vi "UpdateConnectionsListbox.vi"(8 "error in (no error)":errorcluster, 10 "Connections":T1[](array[typedef]), 11 "TCP_serverGUI in":refnum<class "TCP_serverGUI.lvclass">) -> (0 "error out":errorcluster, 3 "TCP_serverGUI out":refnum<class "TCP_serverGUI.lvclass">)   [LabVIEW 2023, in "TCP_serverGUI.lvlib" / "TCP_serverGUI.lvclass"]
uses:
  TCP_serverGUI.lvclass
  TCP_Listener/TypeDefinitions/ConnectionInformation.ctl
  TCP_serverGUI.lvclass/TCP_serverGUI.ctl
  TCP_Listener/TCP_Listener.lvlib
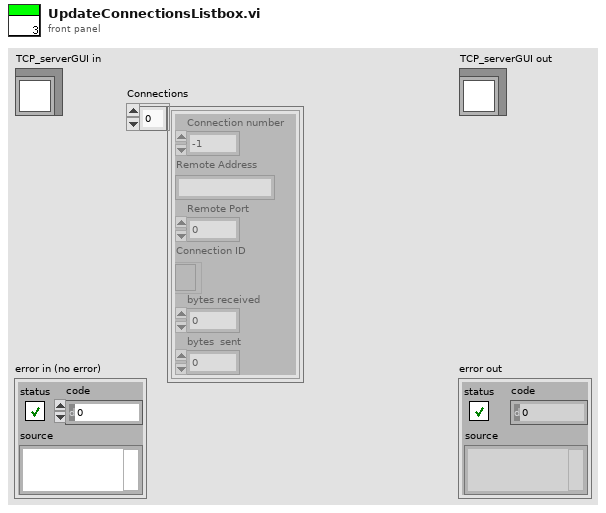
[diagram p1: front panel]
types:
  T1 = typedef "TCP_Listener.lvlib/ConnectionInformation.ctl" = cluster{"Connection number":i32, "Remote Address":string, "Remote Port":u16, "Connection ID":refnum<k5>, "bytes received":i32, "bytes  sent":i32}
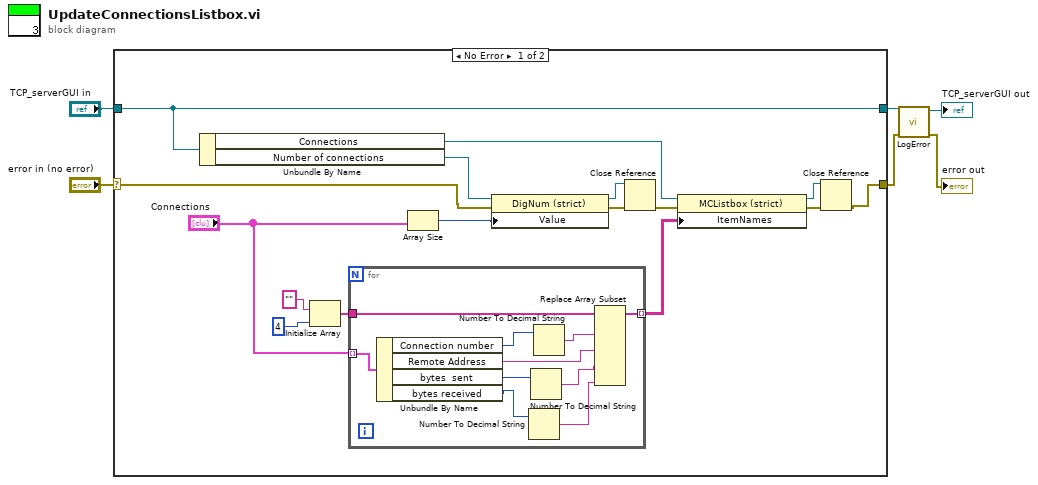
[diagram p0: block diagram]
diagram:
  n1 = case shown="No Error" "error in (no error)" {
    selector: "error in (no error)" -> [w8 w34]
    tunnel: [w7 w34] -> w2
    tunnel: [w22 w33] -> w4
    tunnel: "TCP_serverGUI in" -> [w22 w33]
    frame No Error {
      n2 = Unbundle By Name(w22) -> ("Connections"=w16:refnum<vi>, "Number of connections"=w21:refnum<vi>)
      n3 = Initialize Array("", 4 ("dimension size")) -> (w11:string[])
      n4 = for {
        tunnel: "Connections" -> [w32] mode=indexing
        tunnel: w11 -> [w30]
        tunnel: [w27] -> w9 mode=indexing
        n5 = Unbundle By Name(w32) -> ("Connection number"=w31:i32, "Remote Address"=w28:string, "bytes  sent"=w26:i32, "bytes received"=w25:i32)
        n6 = Number To Decimal String(number=w25) -> (decimal integer string=w23:string)  [unwired: 1 in]
        n7 = Number To Decimal String(number=w26) -> (decimal integer string=w24:string)  [unwired: 1 in]
        n8 = Number To Decimal String(number=w31) -> (decimal integer string=w29:string)  [unwired: 1 in]
        n9 = Replace Array Subset(array=w30, new element #1=w29, new element #2=w28, new element #3=w24, new element #4=w23) -> (w27:string[])  [unwired: 4 in]
      }
      n10 = Array Size(array="Connections") -> (size(s)=w20:i32)
      n11 = property class="DigNum (strict)"(reference=w21, error in=w8, "Value"=w20) -> (reference out=w18:refnum<vi>, error out=w19:errorcluster)
      n12 = Close Reference(reference=w18, error in (no error)=w19) -> (error out=w17:errorcluster)
      n13 = property class="MCListbox (strict)"(reference=w16, error in=w17, "ItemNames"=w9) -> (reference out=w14:refnum<vi>, error out=w15:errorcluster)
      n14 = Close Reference(reference=w14, error in (no error)=w15) -> (error out=w7:errorcluster)
    }
    frame Error {
    }
  }
  n15 = call "LogError.vi"("error in (no error)"=w2, "TCP_serverGUI in"=w4) -> ("error out"=→"error out":errorcluster, "TCP_serverGUI out"=→"TCP_serverGUI out":refnum<class "TCP_serverGUI.lvclass">)  [unwired: 8 in]
